vi "Digital_Bridge_3_kart.vi"() -> ()   [LabVIEW 2014] (continued)
                      }
                      frame True {
                        n1874 = local write "Y1 2"(FALSE ("X1 4")) -> ()
                        n1875 = local write "error"(TRUE ("X1 4")) -> ()
                      }
                    }
                    n1876 = local write "10R Yk"(w4993) -> ()
                    n1877 = local write "output 2 y [10R]"(w4992) -> ()
                  }
                  frame True {
                  }
                }
              }
            }
            n1878 = case shown="True" "read x2 y2 2" {
              frame False {
              }
              frame True {
                n1879 = local read "X Range 10R"() -> (w4827:dbl)
                n1880 = call "only_x_and_y_output.vi"("range"=w4827) -> ("cycle 2"=w4831:bool, "range 2"=w4828:dbl, "Output Y"=w4829:dbl, "Output X"=w4830:dbl)  [unwired: 7 in]
                n1881 = case shown="False" w4831 {
                  tunnel: w4830 -> [w4834 _]
                  tunnel: w4829 -> [w4833 _]
                  tunnel: w4828 -> [w4832 w4842]
                  frame False {
                    n1882 = flat-sequence {
                      tunnel: w4834 -> [w4837]
                      tunnel: w4833 -> [w4836]
                      tunnel: w4832 -> [w4835]
                      frame #0 {
                        n1883 = local write "Output X2"(w4837) -> ()
                        n1884 = local write "Output Y2"(w4836) -> ()
                        n1885 = local write "X Range 10R"(w4835) -> ()
                      }
                      frame #1 {
                        n1886 = global write "DB_Global_4_kart-Test.vi" "amplitude 3/0"(0.0) -> ()
                      }
                      frame #2 {
                        n1887 = Wait (ms)(milliseconds to wait=u32 750) -> ()  [unwired: 1 out]
                      }
                      frame #3 {
                        n1888 = local write "result phase 2"(TRUE ("result phase 4")) -> ()
                        n1889 = local write "read x2 y2 2"(FALSE ("output y")) -> ()
                      }
                    }
                  }
                  frame True {
                    n1890 = local write "X Range 10R"(w4842) -> ()
                  }
                }
              }
            }
            n1891 = case shown="True" "IF ELSE X 2" {
              frame False {
              }
              frame True {
                n1892 = local read "input 1 x [10R]"() -> (w5038:dbl)
                n1893 = local read "input 2 x [10R]"() -> (w5039:dbl)
                n1894 = local read "output 1 x [10R]"() -> (w5042:dbl)
                n1895 = local read "result output x [10R]"() -> (w5044:dbl)
                n1896 = local read "output 2 x [10R]"() -> (w5043:dbl)
                n1897 = call "If Else X.vi"("denge degeri"=2.0, "Xk"=w5038, "X(k-1)"=w5039, "output x 1"=w5042, "output x 2"=w5043, "result output x"=w5044) -> ("Output X(k-1)"=w5037:dbl, "Start X"=w5040:bool)  [unwired: 8 in]
                n1898 = local write "10R X(k-1)"(w5037) -> ()
                n1899 = case shown="True" w5040 {
                  frame False {
                  }
                  frame True {
                    n1900 = local read "count meas"() -> (w5045:u16)
                    n1901 = local write "RESET SENS X 2"(TRUE ("START X 4")) -> ()
                    n1902 = local write "IF ELSE X 2"(FALSE ("IF ELSE X 4")) -> ()
                    n1903 = Increment(x=w5045) -> (x+1=w5046:u16)
                    n1904 = local write "count meas"(w5046) -> ()
                  }
                }
              }
            }
            n1905 = case shown="True" "IF ELSE Y 2" {
              frame False {
              }
              frame True {
                n1906 = local read "input 1 y [10R]"() -> (w4953:dbl)
                n1907 = local read "input 2 y [10R]"() -> (w4954:dbl)
                n1908 = local read "output 1 y [10R]"() -> (w4957:dbl)
                n1909 = local read "result output y [10R]"() -> (w4959:dbl)
                n1910 = local read "output 2 y [10R]"() -> (w4958:dbl)
                n1911 = call "If Else Y.vi"("denge degeri"=2.0, "Yk"=w4953, "Y(k-1)"=w4954, "output y 1"=w4957, "output y 2"=w4958, "result output y"=w4959) -> ("Output Y(k-1)"=w4952:dbl, "Start Y"=w4955:bool)  [unwired: 8 in]
                n1912 = local write "10R Y(k-1)"(w4952) -> ()
                n1913 = case shown="True" w4955 {
                  frame False {
                  }
                  frame True {
                    n1914 = local read "count meas"() -> (w4960:u16)
                    n1915 = local write "RESET SENS Y 2"(TRUE ("START X 4")) -> ()
                    n1916 = local write "IF ELSE Y 2"(FALSE ("IF ELSE X 4")) -> ()
                    n1917 = Increment(x=w4960) -> (x+1=w4961:u16)
                    n1918 = local write "count meas"(w4961) -> ()
                  }
                }
              }
            }
            n1919 = case shown="True" "KONTROL X 2" {
              frame False {
              }
              frame True {
                n1920 = local read "Output Denge Kosulu x1_x2"() -> (w4936:dbl[][])
                n1921 = local read "iterasyon 10R"() -> (w4928:dbl)
                n1922 = local read "Manuel/Otomatik"() -> (w4935:enum16{"Manuel", "Otomatik"})
                n1923 = local read "frekans index"() -> (w4929:dbl)
                n1924 = call "Kontrol X.vi"("denge degeri"=2.0, "İterasyon Denge"=w4928, "Denge Kosulu x1_x2"=w4936, "Manuel/Otomatik"=w4935, "frekans index"=w4929) -> ("Denge Seçimi"=w4932:u8, "New İterasyon Denge"=w4931:dbl, "Iterasyon Count Successful"=w4930:dbl, "Start Denge X"=w4933:bool)  [unwired: 7 in]
                n1925 = case shown="True" w4933 {
                  tunnel: w4932 -> [w4948 _]
                  tunnel: w4931 -> [_ _]
                  tunnel: w4930 -> [w4947 _]
                  frame False {
                    n1926 = local write "Iterasyon Successful"(w4947) -> ()
                    n1927 = local write "1R switch"(TRUE ("10R switch")) -> ()
                    n1928 = local write "Denge Seçimi"(w4948) -> ()
                    n1929 = local read "iterasyon 10R"() -> (w4938:dbl)
                    n1930 = local write "KONTROL X 2"(FALSE ("KONTROL X 2")) -> ()
                    n1931 = local write "Boolean 2"(TRUE ("Boolean 4")) -> ()
                    n1932 = Increment(x=w4938) -> (x+1=w4937:dbl)
                    n1933 = local write "iterasyon 10R"(w4937) -> ()
                    n1934 = local read "cycle 10r 1r"() -> (w4940:bool[])
                    n1935 = local write "count meas"(u16 0 ("count meas")) -> ()
                    n1936 = Replace Array Subset(array=w4940, new element=TRUE ("new element/subarray"), index=0) -> (w4941:bool[])
                    n1937 = local write "cycle 10r 1r"(w4941) -> ()
                  }
                  frame True {
                    n1938 = local write "KONTROL X 2"(FALSE ("KONTROL X 2")) -> ()
                    n1939 = local write "count meas"(u16 0 ("count meas")) -> ()
                    n1940 = local write "RESET SENS X 2"(TRUE ("Start Wagner Y")) -> ()
                  }
                }
              }
            }
            n1941 = case shown="True" "result phase 2" {
              frame False {
              }
              frame True {
                n1942 = flat-sequence {
                  tunnel: [w4872] -> w4867
                  tunnel: w4867 -> [w4888]
                  tunnel: [w4888] -> w4866
                  tunnel: w4866 -> [w4893]
                  tunnel: [w4893] -> w4865
                  tunnel: w4865 -> [w4899]
                  frame #0 {
                    # "pi"
                    n1943 = local read "Output X1"() -> (w4871:dbl)
                    n1944 = local read "Output X2"() -> (w4870:dbl)
                    n1945 = local read "Output Y1"() -> (w4869:dbl)
                    n1946 = local read "Output Y2"() -> (w4868:dbl)
                    n1947 = local read "GPIB In"() -> (w4877:refnum<visa-resource-name>)
                    n1948 = call "return phase.vi"("VISA resource name"=w4877) -> ("return phase"=w4873:string)  [unwired: 10 in]
                    n1949 = Fract/Exp String To Number(use system decimal point (T)=FALSE, string=w4873) -> (number=w4875:dbl)  [unwired: 2 in, 1 out]
                    n1950 = formula code="theta = atan((y2-y1)/(x2-x1))*(180/pi)+phase;"("x1"=w4871, "x2"=w4870, "y1"=w4869, "y2"=w4868, "phase"=w4875, "pi"=3.141592653589793) -> ("theta"=w4872:dbl)
                  }
                  frame #1 {
                    n1951 = local read "frekans index"() -> (w4885:dbl)
                    n1952 = local read "Frekanslar"() -> (w4886:dbl[])
                    n1953 = local read "Direnc 1 - Direnc 2"() -> (w4890:u32)
                    n1954 = property on="Default Values Listbox" class="LstBox (strict)"() -> ("Item Names"=w4887:string[])  [unwired: 2 in, 2 out]
                    n1955 = Fract/Exp String To Number(string=w4887) -> (number=w4884:dbl[])  [unwired: 3 in, 1 out]
                    n1956 = local read "Cluster 2"() -> (w4880:T1)
                    n1957 = Index Array(array=w4886, index=w4885) -> (element=w4882:dbl)
                    n1958 = local read "10R F/P Array"() -> (w4891:dbl[][])
                    n1959 = Search 1D Array(1D array=w4884, element=w4882, start index (0)=0) -> (index of element=w4881:i32)
                    n1960 = Increment(x=w4890) -> (x+1=w4889:u32)
                    n1961 = Replace Array Subset(array=w4891, new element=w4888, index (row)=w4889, index (col)=w4881) -> (w4878:dbl[][])
                    n1962 = local write "10R F/P Array"(w4878) -> ()
                    n1963 = Bundle By Name(cluster=w4880, "10R F/P Array"=w4878) -> (w4879:T1)
                    n1964 = local write "Cluster 2"(w4879) -> ()
                  }
                  frame #2 {
                    n1965 = Wait (ms)(milliseconds to wait=u32 250) -> ()  [unwired: 1 out]
                  }
                  frame #3 {
                    w4896 = u16 0 items=["A", "A-B"] ("Input Source (0: A)")
                    n1966 = local read "GPIB In"() -> (w4895:refnum<visa-resource-name>)
                    n1967 = Number To Fractional String(number=w4899) -> (F-format string=w4900:string)  [unwired: 3 in]
                    n1968 = Search and Replace String(input string=w4900, search string=",", replace string="." ("replace string (\"\")")) -> (result string=w4894:string)  [unwired: 5 in, 3 out]
                    n1969 = call "reference phase.vi"("Reference Phase (0.000 degrees)"=w4894, "VISA resource name"=w4895) -> ("error out"=w4897:errorcluster, "VISA resource name out"=w4898:refnum<visa-resource-name>)  [unwired: 8 in]
                    n1970 = call "input source.vi"("error in (no error)"=w4897, "Input Source (0: A)"=w4896, "VISA resource name"=w4898) -> ()  [unwired: 7 in, 2 out]
                  }
                  frame #4 {
                    n1971 = local write "Contiune 10R"(TRUE ("Contiune Wagner")) -> ()
                    n1972 = local write "result phase 2"(FALSE ("result phase 4")) -> ()
                  }
                }
              }
            }
            n1973 = case shown="True" "KONTROL Y 2" {
              frame False {
              }
              frame True {
                n1974 = local read "Outpu Denge Kosulu y1_y2"() -> (w5021:dbl[][])
                n1975 = local read "iterasyon 10R"() -> (w5013:dbl)
                n1976 = local read "Manuel/Otomatik"() -> (w5020:enum16{"Manuel", "Otomatik"})
                n1977 = local read "frekans index"() -> (w5014:dbl)
                n1978 = call "Kontrol Y.vi"("denge degeri"=2.0, "İterasyon Denge"=w5013, "Denge Kosulu y1_y2"=w5021, "Manuel/Otomatik"=w5020, "frekans index"=w5014) -> ("Denge Seçimi"=w5017:u8, "New İterasyon Denge"=w5016:dbl, "Iterasyon Count Successful"=w5015:dbl, "Start Denge Y"=w5018:bool)  [unwired: 7 in]
                n1979 = case shown="True" w5018 {
                  tunnel: w5017 -> [w5033 _]
                  tunnel: w5016 -> [_ _]
                  tunnel: w5015 -> [w5032 _]
                  frame False {
                    n1980 = local read "iterasyon 10R"() -> (w5023:dbl)
                    n1981 = local write "Iterasyon Successful"(w5032) -> ()
                    n1982 = local write "Denge Seçimi"(w5033) -> ()
                    n1983 = local write "1R switch"(TRUE ("10R switch")) -> ()
                    n1984 = local write "KONTROL Y 2"(FALSE ("KONTROL Y 2")) -> ()
                    n1985 = local write "Boolean 2"(TRUE ("Boolean 4")) -> ()
                    n1986 = Increment(x=w5023) -> (x+1=w5022:dbl)
                    n1987 = local write "iterasyon 10R"(w5022) -> ()
                    n1988 = local read "cycle 10r 1r"() -> (w5025:bool[])
                    n1989 = local write "count meas"(u16 0 ("count meas")) -> ()
                    n1990 = Replace Array Subset(array=w5025, new element=TRUE ("new element/subarray"), index=0) -> (w5026:bool[])
                    n1991 = local write "cycle 10r 1r"(w5026) -> ()
                  }
                  frame True {
                    n1992 = local write "KONTROL Y 2"(FALSE ("KONTROL Y 2")) -> ()
                    n1993 = local write "count meas"(u16 0 ("count meas")) -> ()
                    n1994 = local write "RESET SENS Y 2"(TRUE ("Start Wagner Y")) -> ()
                  }
                }
              }
            }
          }
          frame 3 {
            # "Bu bölümde, ilgili denge durumunun dengede olup olmadığı kontrol edilir.\n\nEğer denge sağlanmışsa, program doğrudan bir sonraki denge aşamasına geçer.\n\nAyrıca, tüm dengeler başarıyla tamamlanmış ve belirlenen ölçüm sayısına ulaşılmışsa, veriler bu alt program (subVI) aracılığıyla Excel dosyasına aktarılır."
            # "Bu bölümün temel amacı, ölçüm aralığını (range) artırmaktır. Program, cihazdan gelen X ve Y değerlerini okuyarak bu değerlerin belirlenen aralık içinde olup olmadığını kontrol eder. \n\nEğer değerler aralık dışındaysa, aralık tekrar artırılır ve ölçüm yeniden yapılır. \n\nAyrıca, bu süreçte input ve output değerleri global değişkenlere kaydedilir. Çünkü sonraki turda, bu kaydedilen değerler farklı bir ölçüm aralığında eğim hesaplaması için kullanılacaktır."
            # "Bu bölümde, sıfırlanacak değer cihazdan okunur. Eğer okunan değer denge koşulunu sağlıyorsa, program Kontrol Y Case’ine geçer. \n\nAncak denge koşulu sağlanmazsa, program if-else yapısına yönlendirilir ve buna göre işlem devam eder."
            # "Bu bölümde, cihaza ikinci input değeri uygulanır ve karşılık gelen output değeri okunur. Daha sonra, hem input hem de output değerleri bir formüle yerleştirilir. Bu formül sayesinde, cihazın 0’a eşitleyeceği (sıfırlayacağı) yeni bir input değeri hesaplanır ve bu değer cihaza uygulanır."
            # "Bu bölümde ilk olarak giriş (input) değeri sisteme uygulanır. Eğer program ilk kez çalıştırılıyorsa, global input üzerinden belirlenen ilk değer (genellikle 0 V) kullanılır. \n\nArdından, cihazdan X değerleri okunur. Bu işlem 10 kez tekrarlanır ve elde edilen ölçümlerin ortalaması alınarak bir sonuç değeri elde edilir. Bu ortalama değer, daha sonra yapılacak işlemlerde kullanılmak üzere saklanır. Özellikle, formül içinde X değerini sıfırlamak için bu bilgiye ihtiyaç duyulur. \n\nEğer girilen input değeri 8 V’tan büyükse, bu durum sistem için güvenli olmayabileceğinden program hata (error) verir ve işlemi durdurur."
            # "Auto Phase, Read X1 Y1, Read X2 Y2, Result Phase: \n\nBu bölümler genel olarak faz ölçümü işlemini gerçekleştirir. \n\nİlk olarak, faz değeri 0’a sıfırlanır. Ardından, global input üzerinden belirlenen range (ölçüm aralığı) değeri uygulanır. Bu işlemden sonra yine global input’ta tanımlanmış olan: \n\nInput 1 verilir ve okuma yapılır (Read X1 Y1) \n\nInput 2 verilir ve okuma yapılır (Read X2 Y2) \n\nBu iki ölçüm sonucuna göre faz değeri bir formül yardımıyla hesaplanır. Elde edilen bu yeni faz değeri, ilgili F/P (frekans/faz) dizisine aktarılır. \n\nBu işlemler, sistemin doğru fazla çalışmasını sağlamak ve sonraki işlemlerde bu bilgiyi referans olarak kullanmak için gerçekleştirilir."
            # "Bu bölümde, Y değerinin dengelendiği kabul edilerek, şimdi sıra X değerinin dengede olup olmadığını kontrol etmeye gelir. \n\nEğer X de dengedeyse, program bir sonraki işlem için ilgili switch case’i aktif eder. \n\nAncak Y dengede değilse, program X’i dengelemeye yönelik işlemlere yönlendirilir."
            # "Bu bölümde, X değerinin dengelendiği kabul edilerek, şimdi sıra Y değerinin dengede olup olmadığını kontrol etmeye gelir. \n\nEğer Y de dengedeyse, program bir sonraki işlem için ilgili switch case’i aktif eder. \n\nAncak Y dengede değilse, program Y’yi dengelemeye yönelik işlemlere yönlendirilir."
            # "X1 3 ile benzer görevi üstleniyor sadece değerler Y oluyor"
            # "IF ELSE X 3 ile benzer görevi üstleniyor sadece değerler Y oluyor"
            # "X 3 ile benzer görevi üstleniyor sadece değerler Y oluyor"
            # "Range Kontrol X 3 ile benzer görevi üstleniyor sadece değerler Y oluyor"
            # "Bu bölümde, daha önce iterasyon (tekrarlama) yapılıp yapılmadığına bakılarak, programın hangi yöne devam edeceğine karar verilir. \n\nEğer gerekli ise, range kontrolü (ölçüm aralığının uygunluğu) yapılır veya sensitivity ayarlama (cihazın duyarlılığını belirleme) bölümlerine yönlendirilir. Bu sayede sistem, ölçüm koşullarına en uygun şekilde ayarlanarak doğru ve güvenilir sonuçlar elde edilmesi sağlanır."
            # "Bu bölümde, daha önce belirlenen F/P dizilerindeki (frekans/faz değerleri) faz bilgileri, mevcut frekansa göre uygulanır. Ardından, ilgili denge koşulunun daha önce gerçekleştirilip gerçekleştirilmediği kontrol edilir. \nEğer bu denge daha önce sağlanmamışsa, program uygun faz ayarlamasını yapar. Ancak denge daha önce zaten kurulmuşsa, faz ayarı yapılmadan işleme devam edilir. Bu sayede gereksiz tekrarların önüne geçilmiş olur."
            # "Bu bölümde öncelikle, sistemin kaç kez ölçüm yaptığına işaret eden meas number (ölçüm sayısı) kontrol edilir. \nEğer bu sayı 6’dan büyükse (bu sınır kullanıcı tarafından belirlenmiştir ve değiştirilebilir), program hata verir ve reset values adlı bölüme yönlenir. Bu durum, sistemin çok fazla başarısız deneme yapmasını engellemek içindir. \nEğer ölçüm sayısı 6’dan küçükse, program global bir değişken olan sensitivity (duyarlılık) değerini ayarlar ve ardından işlemlere devam etmek üzere Start X bölümüne geçer."
            # "Bu bölümde, ölçüm için gerekli olan giriş (input) değerleri sisteme girilir. Girişler tamamlandıktan sonra program, ölçüm işlemini başlatmak üzere X adlı bölüme yönlendirilir. Bu adım, ölçüm sürecinin fiilen başlatıldığı ilk noktadır."
            # "Pass subvi girmeden önce doğru range miyiz değil miyiz ölçüyor, değil ise +2 üst kademeye gidiyor"
            # "Start 1R X ile benzer görevi üstleniyor sadece değerler Y oluyor"
            # "Reset Sens X 3 ile benzer görevi üstleniyor sadece değerler Y oluyor"
            # "Start X 3 ile benzer görevi üstleniyor sadece değerler Y oluyor"
            # "Bu bölüm, iterasyona (tekrarlamalı işleme) bağlı olarak Reserve ayarının maksimumda mı yoksa minimumda mı olacağını belirler. Aynı zamanda, ölçüm sürecinin başlangıcında kullanılacak olan sensitivity  değerleri de bu bölümde ayarlanır. Bu ayarlar, ölçüm sırasında cihazın hassasiyetini ve çalışma aralığını doğru şekilde belirlemek için gereklidir."
            # "1R"
            n1995 = case shown="True" "Start 1R Y" {
              frame False {
              }
              frame True {
                n1996 = flat-sequence {
                  frame #0 {
                    w5867 = u16 0 items=["A", "A-B"] ("Input Source (0: A)")
                    n1997 = local read "frekans index"() -> (w5861:dbl)
                    n1998 = local read "Frekanslar"() -> (w5862:dbl[])
                    n1999 = local read "Direnc 1 - Direnc 2"() -> (w5864:u32)
                    n2000 = local read "1R F/P Array"() -> (w5865:dbl[][])
                    n2001 = Index Array(array=w5862, index=w5861) -> (element=w5863:dbl)
                    n2002 = call "get_phase_element.vi"("index r"=w5864, "hz"=w5863, "Array"=w5865) -> ("element"=w5857:dbl)  [unwired: 8 in]
                    n2003 = Number To Fractional String(number=w5857) -> (F-format string=w5858:string)  [unwired: 3 in]
                    n2004 = Search and Replace String(input string=w5858, search string=",", replace string="." ("replace string (\"\")")) -> (result string=w5856:string)  [unwired: 5 in, 3 out]
                    n2005 = local read "GPIB In"() -> (w5866:refnum<visa-resource-name>)
                    n2006 = call "reference phase.vi"("Reference Phase (0.000 degrees)"=w5856, "VISA resource name"=w5866) -> ("error out"=w5868:errorcluster, "VISA resource name out"=w5869:refnum<visa-resource-name>)  [unwired: 8 in]
                    n2007 = call "input source.vi"("error in (no error)"=w5868, "Input Source (0: A)"=w5867, "VISA resource name"=w5869) -> ()  [unwired: 7 in, 2 out]
                  }
                  frame #1 {
                    n2008 = local write "Boolean 3"(FALSE ("Boolean 4")) -> ()
                    n2009 = local write "Start 1R Y"(FALSE ("START Y 6")) -> ()
                    n2010 = local write "RESET SENS Y 3"(TRUE ("START X")) -> ()
                  }
                }
              }
            }
            n2011 = case shown="True" "RESET SENS Y 3" {
              frame False {
              }
              frame True {
                n2012 = local read "count meas"() -> (w5836:u16)
                n2013 = local read "iterasyon 1R"() -> (w5834:dbl)
                n2014 = Greater?(x=w5836, y=u16 8) -> (0:w5833:bool)
                n2015 = Greater?(x=w5834, y=10.0) -> (0:w5832:bool)
                n2016 = Or(x=w5833, y=w5832) -> (x .or. y?=w5831:bool)
                n2017 = case shown="True" w5831 {
                  frame False {
                    n2018 = flat-sequence {
                      frame #0 {
                        n2019 = global read "show_sensitivity.vi" "show sensitivity (1R  y)"() -> (w5838:dbl)
                        n2020 = local read "GPIB In"() -> (w5839:refnum<visa-resource-name>)
                        n2021 = call "get_sensitivity.vi"("input 1"=w5838, "SR850 GPIB In"=w5839) -> ()  [unwired: 8 in, 2 out]
                      }
                      frame #1 {
                        n2022 = Wait (ms)(milliseconds to wait=u32 500) -> ()  [unwired: 1 out]
                      }
                      frame #2 {
                        n2023 = local write "RESET SENS Y 3"(FALSE ("RESET SENS X")) -> ()
                        n2024 = local write "START Y 3"(TRUE ("START X 4")) -> ()
                      }
                    }
                  }
                  frame True {
                    n2025 = local read "iterasyon 1R"() -> (w5845:dbl)
                    n2026 = Greater?(x=w5845, y=10.0) -> (0:w5843:bool)
                    n2027 = case shown="False" w5843 {
                      frame False {
                        n2028 = flat-sequence {
                          frame #0 {
                            n2029 = local write "RESET SENS Y 3"(FALSE ("Start 10R X")) -> ()
                            n2030 = local write "İterasyon X 3"(0.0 ("İterasyon X 3")) -> ()
                            n2031 = local write "count meas"(u16 9 ("count meas")) -> ()
                          }
                          frame #1 {
                            n2032 = local write "reset values"(TRUE ("Start 10R X")) -> ()
                            n2033 = local write "error"(TRUE ("Start 10R X")) -> ()
                          }
                        }
                      }
                      frame True {
                        n2034 = flat-sequence {
                          frame #0 {
                            n2035 = local write "RESET SENS Y 3"(FALSE ("Start 10R X")) -> ()
                            n2036 = local write "İterasyon X 3"(0.0 ("İterasyon X 3")) -> ()
                            n2037 = local write "count meas"(u16 10 ("count meas")) -> ()
                          }
                          frame #1 {
                            n2038 = local write "reset values"(TRUE ("Start 10R X")) -> ()
                            n2039 = local write "error"(TRUE ("Start 10R X")) -> ()
                          }
                        }
                      }
                    }
                  }
                }
              }
            }
            n2040 = case shown="True" "START Y 3" {
              frame False {
              }
              frame True {
                n2041 = flat-sequence {
                  frame #0 {
                    n2042 = local read "1R Y(k-1)"() -> (w5874:dbl)
                    n2043 = local read "1R Yk"() -> (w5873:dbl)
                    n2044 = local write "input 1 y [1R]"(w5873) -> ()
                    n2045 = local write "input 2 y [1R]"(w5874) -> ()
                    n2046 = global write "DB_Global_4_kart-Test.vi" "phase 3/1"(w5873) -> ()
                  }
                  frame #1 {
                    n2047 = Wait (ms)(milliseconds to wait=u32 500) -> ()  [unwired: 1 out]
                  }
                  frame #2 {
                    n2048 = local write "START Y 3"(FALSE ("START X")) -> ()
                    n2049 = local write "Y 3"(TRUE ("START X")) -> ()
                  }
                }
              }
            }
            n2050 = case shown="True" "Start 1R X" {
              frame False {
              }
              frame True {
                n2051 = flat-sequence {
                  frame #0 {
                    w5774 = u16 0 items=["A", "A-B"] ("Input Source (0: A)")
                    n2052 = local read "frekans index"() -> (w5769:dbl)
                    n2053 = local read "Frekanslar"() -> (w5770:dbl[])
                    n2054 = local read "Direnc 1 - Direnc 2"() -> (w5771:u32)
                    n2055 = local read "1R F/P Array"() -> (w5772:dbl[][])
                    n2056 = Index Array(array=w5770, index=w5769) -> (element=w5768:dbl)
                    n2057 = call "get_phase_element.vi"("index r"=w5771, "hz"=w5768, "Array"=w5772) -> ("element"=w5764:dbl)  [unwired: 8 in]
                    n2058 = Number To Fractional String(number=w5764) -> (F-format string=w5767:string)  [unwired: 3 in]
                    n2059 = local read "GPIB In"() -> (w5773:refnum<visa-resource-name>)
                    n2060 = Search and Replace String(input string=w5767, search string=",", replace string="." ("replace string (\"\")")) -> (result string=w5763:string)  [unwired: 5 in, 3 out]
                    n2061 = call "reference phase.vi"("Reference Phase (0.000 degrees)"=w5763, "VISA resource name"=w5773) -> ("error out"=w5775:errorcluster, "VISA resource name out"=w5776:refnum<visa-resource-name>)  [unwired: 8 in]
                    n2062 = call "input source.vi"("error in (no error)"=w5775, "Input Source (0: A)"=w5774, "VISA resource name"=w5776) -> ()  [unwired: 7 in, 2 out]
                  }
                  frame #1 {
                    n2063 = local read "1 or 10"() -> (w5791:i32)
                    n2064 = local read "İterasyon X 3"() -> (w5787:dbl)
                    n2065 = local read "frekans index"() -> (w5786:dbl)
                    n2066 = local read "control hz array"() -> (w5782:dbl[][])
                    n2067 = Greater?(x=w5787, y=0.0) -> (0:w5788:bool)
                    n2068 = call "change2d.vi"("reset(default false)"=FALSE, "index (col)"=w5786, "index (row)"=2, "read/write(T/F)"=TRUE, "2D Array"=w5782) -> ("result count"=w5781:dbl)  [unwired: 5 in, 1 out]
                    n2069 = Equal?(x=w5791, y=1) -> (x = y?=w5789:bool)
                    n2070 = Or(x=w5788, y=w5789) -> (x .or. y?=w5778:bool)
                    n2071 = local read "set"() -> (w5780:u16)
                    n2072 = Equal?(x=w5781, y=w5780) -> (x = y?=w5779:bool)
                    n2073 = Or(x=w5778, y=w5779) -> (x .or. y?=w5777:bool)
                    n2074 = case shown="True" w5777 {
                      frame False {
                        n2075 = local write "auto phase 1R"(TRUE ("auto phase 10R")) -> ()
                        n2076 = local write "Start 1R X"(FALSE ("auto phase 10R")) -> ()
                      }
                      frame True {
                        n2077 = local write "Contiune 1R"(TRUE) -> ()
                        n2078 = local write "Start 1R X"(FALSE ("START WAGNER")) -> ()
                      }
                    }
                  }
                }
              }
            }
            n2079 = case shown="True" "1R switch" {
              frame False {
              }
              frame True {
                n2080 = flat-sequence {
                  frame #0 {
                    n2081 = local read "iterasyon 1R"() -> (w5797:dbl)
                    n2082 = Equal?(x=w5797, y=0.0) -> (x = y?=w5798:bool)
                    n2083 = case shown="True" w5798 {
                      frame False {
                      }
                      frame True {
                        n2084 = local read "1 or 10"() -> (w5800:i32)
                        n2085 = case shown="1" w5800 {
                          frame 0, Default {
                          }
                          frame 1 {
                            n2086 = local write "iterasyon 1R"(1.0 ("iterasyon WAGNER")) -> ()
                          }
                        }
                      }
                    }
                  }
                  frame #1 {
                    n2087 = local read "iterasyon 1R"() -> (w5803:dbl)
                    n2088 = Greater?(x=w5803, y=0.0) -> (0:w5802:bool)
                    n2089 = case shown="True" w5802 {
                      frame False {
                        n2090 = local read "Reserve 1R"() -> (w5806:u16)
                        n2091 = case shown="0, Default" w5806 {
                          tunnel: ["0" ("Reserve(MAX-MIN)") "1" ("Reserve(MAX-MIN)") "2" ("Reserve(MAX-MIN)")] -> w5805
                          frame 0, Default {
                          }
                          frame 1 {
                          }
                          frame 2 {
                          }
                        }
                        n2092 = local read "GPIB In"() -> (w5807:refnum<visa-resource-name>)
                        n2093 = call "Reserve.vi"("Reserve(MAX-MIN)"=w5805, "VISA resource name"=w5807) -> ()  [unwired: 8 in, 2 out]
                      }
                      frame True {
                        n2094 = local read "GPIB In"() -> (w5812:refnum<visa-resource-name>)
                        n2095 = call "Reserve.vi"("Reserve(MAX-MIN)"="0", "VISA resource name"=w5812) -> ()  [unwired: 8 in, 2 out]
                      }
                    }
                  }
                  frame #2 {
                    n2096 = Wait (ms)(milliseconds to wait=u32 500) -> ()  [unwired: 1 out]
                  }
                  frame #3 {
                    w5815 = u16 1 items=["Wagner", "Ground"] ("Switch")
                    w5816 = u16 3 items=["Open All", "Ana Denge", "10R", "1R"] ("Ring")
                    n2097 = call "mux1.vi"("Ring"=w5816) -> ("error out"=w5817:errorcluster)  [unwired: 9 in]
                    n2098 = property on="Tab Control" class="TabCtl (strict)"("Value"=T4."1R" ("Tab Control")) -> ()  [unwired: 2 in, 2 out]
                    n2099 = call "mux2.vi"("Switch"=w5815, "error in (no error)"=w5817) -> ()  [unwired: 6 in, 1 out]
                  }
                  frame #4 {
                    n2100 = Wait (ms)(milliseconds to wait=u32 1000) -> ()  [unwired: 1 out]
                  }
                  frame #5 {
                    n2101 = local read "İterasyon X 3"() -> (w5825:dbl)
                    n2102 = local read "1 or 10"() -> (w5822:i32)
                    n2103 = Equal?(x=w5822, y=1) -> (x = y?=w5821:bool)
                    n2104 = Greater?(x=w5825, y=0.0) -> (0:w5820:bool)
                    n2105 = Or(x=w5820, y=w5821) -> (x .or. y?=w5819:bool)
                    n2106 = case shown="False" w5819 {
                      frame False {
                        n2107 = local read "X Range 1R"() -> (w5827:dbl)
                        n2108 = local read "Y Range 1R"() -> (w5826:dbl)
                        n2109 = global write "show_sensitivity.vi" "show sensitivity (1R  x)"(w5827) -> ()
                        n2110 = global write "show_sensitivity.vi" "show sensitivity (1R  y)"(w5826) -> ()
                      }
                      frame True {
                        w5828 = 16.0 ("Max. Hassasiyet")
                        n2111 = global write "show_sensitivity.vi" "show sensitivity (1R  x)"(w5828) -> ()
                        n2112 = global write "show_sensitivity.vi" "show sensitivity (1R  y)"(w5828) -> ()
                      }
                    }
                  }
                  frame #6 {
                    n2113 = local write "Start 1R X"(TRUE ("START WAGNER")) -> ()
                    n2114 = local write "1R switch"(FALSE ("wagner switch")) -> ()
                  }
                }
              }
            }
            n2115 = case shown="True" "RESET SENS X 3" {
              frame False {
              }
              frame True {
                n2116 = local read "count meas"() -> (w5884:u16)
                n2117 = local read "iterasyon 1R"() -> (w5881:dbl)
                n2118 = Greater?(x=w5884, y=u16 8) -> (0:w5880:bool)
                n2119 = Greater?(x=w5881, y=5.0) -> (0:w5879:bool)
                n2120 = Or(x=w5880, y=w5879) -> (x .or. y?=w5878:bool)
                n2121 = case shown="True" w5878 {
                  frame False {
                    n2122 = flat-sequence {
                      frame #0 {
                        n2123 = global read "show_sensitivity.vi" "show sensitivity (1R  x)"() -> (w5885:dbl)
                        n2124 = local read "GPIB In"() -> (w5886:refnum<visa-resource-name>)
                        n2125 = call "get_sensitivity.vi"("input 1"=w5885, "SR850 GPIB In"=w5886) -> ()  [unwired: 8 in, 2 out]
                      }
                      frame #1 {
                        n2126 = Wait (ms)(milliseconds to wait=u32 500) -> ()  [unwired: 1 out]
                      }
                      frame #2 {
                        n2127 = local write "RESET SENS X 3"(FALSE ("RESET SENS X")) -> ()
                        n2128 = local write "START X 3"(TRUE ("START X 4")) -> ()
                      }
                    }
                  }
                  frame True {
                    n2129 = local read "iterasyon 1R"() -> (w5892:dbl)
                    n2130 = Greater?(x=w5892, y=5.0) -> (0:w5890:bool)
                    n2131 = case shown="False" w5890 {
                      frame False {
                        n2132 = flat-sequence {
                          frame #0 {
                            n2133 = local write "count meas"(u16 9 ("count meas")) -> ()
                            n2134 = local write "İterasyon X 3"(0.0 ("İterasyon X 3")) -> ()
                            n2135 = local write "RESET SENS X 3"(FALSE ("Start 10R X")) -> ()
                          }
                          frame #1 {
                            n2136 = local write "reset values"(TRUE ("Start 10R X")) -> ()
                            n2137 = local write "error"(TRUE ("Start 10R X")) -> ()
                          }
                        }
                      }
                      frame True {
                        n2138 = flat-sequence {
                          frame #0 {
                            n2139 = local write "count meas"(u16 10 ("count meas")) -> ()
                            n2140 = local write "İterasyon X 3"(0.0 ("İterasyon X 3")) -> ()
                            n2141 = local write "RESET SENS X 3"(FALSE ("Start 10R X")) -> ()
                          }
                          frame #1 {
                            n2142 = local write "reset values"(TRUE ("Start 10R X")) -> ()
                            n2143 = local write "error"(TRUE ("Start 10R X")) -> ()
                          }
                        }
                      }
                    }
                  }
                }
              }
            }
            n2144 = case shown="True" "START X 3" {
              frame False {
              }
              frame True {
                n2145 = flat-sequence {
                  frame #0 {
                    n2146 = local read "1R X(k-1)"() -> (w5904:dbl)
                    n2147 = local read "1R Xk"() -> (w5903:dbl)
                    n2148 = global write "DB_Global_4_kart-Test.vi" "amplitude 3/1"(w5903) -> ()
                    n2149 = local write "input 1 x [1R]"(w5903) -> ()
                    n2150 = local write "input 2 x [1R]"(w5904) -> ()
                  }
                  frame #1 {
                    n2151 = Wait (ms)(milliseconds to wait=u32 500) -> ()  [unwired: 1 out]
                  }
                  frame #2 {
                    n2152 = local write "START X 3"(FALSE ("START X 4")) -> ()
                    n2153 = local write "X 3"(TRUE ("START X")) -> ()
                  }
                  frame #3 {
                  }
                }
              }
            }
            n2154 = case shown="True" "Optimum Range 3" {
              frame False {
              }
              frame True {
                n2155 = flat-sequence {
                  frame #0 {
                    n2156 = global read "show_sensitivity.vi" "show sensitivity (1R  x)"() -> (w5417:dbl)
                    n2157 = local read "GPIB In"() -> (w5416:refnum<visa-resource-name>)
                    n2158 = call "get_sensitivity.vi"("input 1"=w5417, "SR850 GPIB In"=w5416) -> ()  [unwired: 8 in, 2 out]
                  }
                  frame #1 {
                    n2159 = call "set optimum range.vi"("denge degeri"=3.0) -> ("ok"=w5418:bool)  [unwired: 14 in]
                    n2160 = case shown="True" w5418 {
                      frame False {
                      }
                      frame True {
                        n2161 = local write "Optimum Range 3"(FALSE ("Optimum Range 1")) -> ()
                        n2162 = local write "PASS 1R"(TRUE ("PASS 1R")) -> ()
                      }
                    }
                  }
                }
              }
            }
            n2163 = case shown="True" "Contiune 1R" {
              frame False {
              }
              frame True {
                n2164 = local read "1 or 10"() -> (w5472:i32)
                n2165 = local read "frekans index"() -> (w5471:dbl)
                n2166 = local read "control hz array"() -> (w5467:dbl[][])
                n2167 = call "change2d.vi"("reset(default false)"=FALSE, "index (col)"=w5471, "index (row)"=2, "read/write(T/F)"=TRUE, "2D Array"=w5467) -> ("result count"=w5466:dbl)  [unwired: 5 in, 1 out]
                n2168 = local read "iterasyon 1R"() -> (w5476:dbl)
                n2169 = local read "set"() -> (w5465:u16)
                n2170 = case shown="1" w5472 {
                  tunnel: [FALSE TRUE] -> w5473
                  frame 10, Default {
                  }
                  frame 1 {
                  }
                }
                n2171 = Equal?(x=w5466, y=w5465) -> (x = y?=w5464:bool)
                n2172 = Greater?(x=w5476, y=0.0) -> (0:w5474:bool)
                n2173 = Or(x=w5474, y=w5473) -> (x .or. y?=w5463:bool)
                n2174 = Or(x=w5463, y=w5464) -> (x .or. y?=w5462:bool)
                n2175 = case shown="True" w5462 {
                  frame False {
                    n2176 = local write "RESET SENS X 3"(TRUE ("START X")) -> ()
                    n2177 = local write "Contiune 1R"(FALSE ("START WAGNER")) -> ()
                    n2178 = local write "Boolean 3"(FALSE ("Boolean 4")) -> ()
                  }
                  frame True {
                    n2179 = local write "Optimum Range 3"(TRUE ("START X")) -> ()
                    n2180 = local write "Contiune 1R"(FALSE ("Boolean 4")) -> ()
                    n2181 = local write "Boolean 3"(FALSE ("Boolean 4")) -> ()
                  }
                }
              }
            }
            n2182 = case shown="True" "PASS 1R" {
              frame False {
              }
              frame True {
                n2183 = flat-sequence {
                  tunnel: [w5664] -> w5654
                  tunnel: [w5663] -> w5653
                  tunnel: [w5662] -> w5652
                  tunnel: [w5661] -> w5651
                  tunnel: [w5660] -> w5650
                  tunnel: [w5659] -> w5649
                  tunnel: [w5658] -> w5648
                  tunnel: w5654 -> [w5726]
                  tunnel: w5653 -> [w5725]
                  tunnel: w5652 -> [w5724]
                  tunnel: w5651 -> [w5723]
                  tunnel: w5650 -> [w5722]
                  tunnel: w5649 -> [w5721]
                  tunnel: w5648 -> [w5720]
                  frame #0 {
                    n2184 = Wait (ms)(milliseconds to wait=u32 500) -> ()  [unwired: 1 out]
                  }
                  frame #1 {
                    n2185 = local read "Other Array"() -> (w5692:dbl[])
                    n2186 = for {
                      N: 7 -> [_]
                      shift-right: [w5709] -> w5695
                      shift-left: w5692 -> [w5712]
                      i -> [w5711]
                      n2187 = case shown="6" w5711 {
                        tunnel: [3.0 ("iterasyon WAGNER") w5714 w5715 w5716 w5717 w5718 w5719] -> w5710
                        frame 0, Default {
                        }
                        frame 1 {
                          n2188 = local read "Iterasyon Successful"() -> (w5714:dbl)
                        }
                        frame 2 {
                          n2189 = local read "Direnc 1 - Direnc 2"() -> (w5715:u32)
                        }
                        frame 3 {
                          n2190 = local read "olcum"() -> (w5716:u16)
                        }
                        frame 4 {
                          n2191 = local read "set"() -> (w5717:u16)
                        }
                        frame 5 {
                          n2192 = local read "frekans index"() -> (w5718:dbl)
                        }
                        frame 6 {
                          n2193 = local read "iterasyon 1R"() -> (w5719:dbl)
                        }
                      }
                      n2194 = Replace Array Subset(array=w5712, new element=w5710, index=w5711) -> (w5709:dbl[])
                    }
                    n2195 = local read "Output Denge Kosulu x2_y2"() -> (w5697:dbl[][])
                    n2196 = local read "Output Denge Kosulu x1_x2"() -> (w5678:dbl[][])
                    n2197 = control-ref of="Default Values Listbox"() -> (w5682:refnum<vi>)
                    n2198 = local read "Outpu Denge Kosulu y1_y2"() -> (w5677:dbl[][])
                    n2199 = local read "Frekanslar"() -> (w5657:dbl[])
                    n2200 = local read "Cluster"() -> (w5680:T2)
                    n2201 = local read "Cluster 2"() -> (w5679:T1)
                    n2202 = Array Size(array=w5657) -> (size(s)=w5656:i32)
                    n2203 = call "merge_x_y.vi"("frekans size"=w5656, "y1_y2"=w5677, "x1_x2"=w5678) -> ("x1_x2_y1_y2"=w5676:dbl[][])  [unwired: 8 in]
                    n2204 = local read "default values"() -> (w5696:T3)
                    n2205 = local read "input values"() -> (w5681:dbl[])
                    n2206 = local read "Sheet name"() -> (w5693:string)
                    n2207 = local read "Other Boolean Array"() -> (w5691:bool[])
                    n2208 = for {
                      N: 5 -> [_]
                      shift-right: [w5700] -> w5694
                      shift-left: w5691 -> [w5703]
                      i -> [w5702]
                      n2209 = case shown="1" w5702 {
                        tunnel: [FALSE FALSE FALSE FALSE FALSE] -> w5701
                        frame 0, Default {
                        }
                        frame 1 {
                        }
                        frame 2 {
                        }
                        frame 3 {
                        }
                        frame 4 {
                        }
                      }
                      n2210 = Replace Array Subset(array=w5703, new element=w5701, index=w5702) -> (w5700:bool[])
                    }
                    n2211 = call "Pass.vi"("Other Array"=w5695, "Other Boolean Array"=w5694, "Denge Kosulu x2_y2"=w5697, "LstBox Refnum"=w5682, "Cluster"=w5680, "F/P Array Cluster"=w5679, "Sheet name"=w5693, "default values"=w5696, "x1_x2_y1_y2"=w5676, "input values"=w5681) -> ("output values"=w5675:dbl[], "Output Other Boolean Array"=w5688:bool[], "Output Cluster"=w5674:T2, "Output F/P Array Cluster"=w5670:T1, "output default values"=w5690:T11, "Output Iterasyon Successful"=w5689:dbl, "Denge Seçimi"=w5662:u8, "end time"=w5660:string)  [unwired: 1 in, 1 out]
                    n2212 = Unbundle By Name(w5674) -> ("F Values Array"=w5673:dbl[][], "control hz array"=w5672:dbl[][], "extra default values"=w5671:dbl[][])
                    n2213 = Unbundle By Name(w5670) -> ("AD F/P Array"=w5669:dbl[][], "10R F/P Array"=w5668:dbl[][], "1R F/P Array"=w5667:dbl[][], "Wagner F/P Array"=w5666:dbl[][], "Kelvin F/P Array"=w5665:dbl[][])
                    n2214 = local write "input values"(w5675) -> ()
                    n2215 = local write "AD F/P Array"(w5669) -> ()
                    n2216 = local write "10R F/P Array"(w5668) -> ()
                    n2217 = local write "1R F/P Array"(w5667) -> ()
                    n2218 = local write "Wagner F/P Array"(w5666) -> ()
                    n2219 = local write "Kelvin F/P Array"(w5665) -> ()
                    n2220 = local write "F Values Array"(w5673) -> ()
                    n2221 = local write "control hz array"(w5672) -> ()
                    n2222 = local write "extra default values"(w5671) -> ()
                    n2223 = local write "default values"(w5690) -> ()
                    n2224 = local write "Iterasyon Successful"(w5689) -> ()
                    n2225 = Index Array(array=w5688, index #1=0 ("index"), index #2=1 ("index"), index #3=2 ("index"), index #4=3 ("index"), index #5=4 ("index")) -> (element #1=w5664:bool, element #2=w5663:bool, element #3=w5661:bool, element #4=w5659:bool, element #5=w5658:bool)
                  }
                  frame #2 {
                    n2226 = case shown="True" w5720 {
                      frame False {
                      }
                      frame True {
                        n2227 = local write "RESET SENS Y 3"(TRUE ("RESET SENS Y 4")) -> ()
                        n2228 = local write "PASS 1R"(FALSE ("PASS 1R")) -> ()
                      }
                    }
                    n2229 = case shown="True" w5726 {
                      frame False {
                      }
                      frame True {
                        n2230 = local write "reset values"(TRUE ("reset values")) -> ()
                        n2231 = local write "PASS 1R"(FALSE ("PASS 1R")) -> ()
                        n2232 = local write "pass hz"(TRUE ("pass hz")) -> ()
                        n2233 = local write "Boolean 3"(TRUE ("Boolean 4")) -> ()
                      }
                    }
                    n2234 = case shown="True" w5725 {
                      tunnel: w5724 -> [_ w5735]
                      frame False {
                      }
                      frame True {
                        n2235 = local read "cycle 10r 1r"() -> (w5738:bool[])
                        n2236 = Index Array(array=w5738, index=0) -> (element=w5736:bool)
                        n2237 = case shown="False" w5736 {
                          tunnel: w5735 -> [_ w5745]
                          frame False {
                            n2238 = local write "Denge Seçimi"(u8 2 ("Denge Seçimi")) -> ()
                            n2239 = local write "count meas"(u16 0 ("count meas")) -> ()
                            n2240 = local write "10R switch"(TRUE ("10R switch")) -> ()
                            n2241 = local write "Boolean 3"(TRUE ("Boolean 4")) -> ()
                            n2242 = local write "PASS 1R"(FALSE ("PASS 1R")) -> ()
                          }
                          frame True {
                            n2243 = local write "Denge Seçimi"(w5745) -> ()
                            n2244 = local write "kelvin switch"(TRUE ("10R switch")) -> ()
                            n2245 = local write "count meas"(u16 0 ("count meas")) -> ()
                            n2246 = local write "Boolean 3"(TRUE ("Boolean 4")) -> ()
                            n2247 = local write "PASS 1R"(FALSE ("PASS 1R")) -> ()
                          }
                        }
                      }
                    }
                    n2248 = case shown="True" w5723 {
                      tunnel: w5722 -> [_ w5733]
                      frame False {
                      }
                      frame True {
                        n2249 = local write "reset values"(TRUE ("reset values")) -> ()
                        n2250 = local write "end time"(w5733) -> ()
                        n2251 = local write "Boolean 3"(TRUE ("Boolean 4")) -> ()
                        n2252 = local write "PASS 1R"(FALSE ("PASS 1R")) -> ()
                      }
                    }
                    n2253 = case shown="True" w5721 {
                      frame False {
                      }
                      frame True {
                        n2254 = local write "RESET SENS X 3"(TRUE ("RESET SENS X 4")) -> ()
                        n2255 = local write "PASS 1R"(FALSE ("PASS 1R")) -> ()
                      }
                    }
                  }
                  frame #3 {
                  }
                }
              }
            }
            n2256 = case shown="True" "auto phase 1R" {
              frame False {
              }
              frame True {
                n2257 = flat-sequence {
                  frame #0 {
                    n2258 = local read "GPIB In"() -> (w5754:refnum<visa-resource-name>)
                    n2259 = call "reference phase.vi"("Reference Phase (0.000 degrees)"="0", "VISA resource name"=w5754) -> ()  [unwired: 8 in, 2 out]
                  }
                  frame #1 {
                    w5756 = u16 0 items=["100 nV", "200 nV", "500 nV", "1 uV", "2 uV", "5 uV", "10 uV", "20 uV", "50 uV", "100 uV", "200 uV", "500 uV", "1 mV"] ("Min. Hassasiyet")
                    n2260 = local read "GPIB In"() -> (w5757:refnum<visa-resource-name>)
                    n2261 = local read "X Range 1R"() -> (w5755:dbl)
                    n2262 = call "GAIN BASIC.vi"("SR850 GPIB In"=w5757, "Max. Hassasiyet"=w5755, "Auto Gain (False)"=FALSE, "Min. Hassasiyet"=w5756) -> ()  [unwired: 10 in, 2 out]
                  }
                  frame #2 {
                    n2263 = local read "X 1.input 1R"() -> (w5759:dbl)
                    n2264 = global write "DB_Global_4_kart-Test.vi" "amplitude 3/1"(w5759) -> ()
                    n2265 = global write "DB_Global_4_kart-Test.vi" "phase 3/1"(w5759) -> ()
                  }
                  frame #3 {
                    n2266 = Wait (ms)(milliseconds to wait=u32 750) -> ()  [unwired: 1 out]
                  }
                  frame #4 {
                    n2267 = local write "read x1 y1 3"(TRUE ("output x")) -> ()
                    n2268 = local write "auto phase 1R"(FALSE ("auto phase wagner")) -> ()
                  }
                }
              }
            }
            n2269 = case shown="True" "RANGE KONTROL X 3" {
              frame False {
              }
              frame True {
                n2270 = local read "Output Denge Kosulu x1_x2"() -> (w5605:dbl[][])
                n2271 = local read "iterasyon 1R"() -> (w5604:dbl)
                n2272 = local read "frekans index"() -> (w5597:dbl)
                n2273 = local read "input 1 x [1R]"() -> (w5606:dbl)
                n2274 = local read "input 2 x [1R]"() -> (w5607:dbl)
                n2275 = local read "output 2 x [1R]"() -> (w5601:dbl)
                n2276 = local read "output 1 x [1R]"() -> (w5603:dbl)
                n2277 = call "Range Kontrol X.vi"("denge degeri"=3.0, "iterasyon Denge"=w5604, "frekans index"=w5597, "Denge Kosulu x1_x2"=w5605, "Xk"=w5606, "X(k-1)"=w5607, "output x 1"=w5603, "output x 2"=w5601) -> ("Output X(k-1)"=w5596:dbl, "result output x"=w5608:dbl, "KONTROL Y"=w5600:bool, "IF ELSE"=w5599:bool, "Start Denge Y"=w5598:bool)  [unwired: 7 in]
                n2278 = local write "1R X(k-1)"(w5596) -> ()
                n2279 = local write "result output x [1R]"(w5608) -> ()
                n2280 = flat-sequence {
                  tunnel: w5600 -> [w5611]
                  tunnel: w5599 -> [w5610]
                  tunnel: w5598 -> [w5609]
                  frame #0 {
                    n2281 = case shown="True" w5609 {
                      frame False {
                      }
                      frame True {
                        n2282 = local write "Start 1R Y"(TRUE ("Start Wagner Y")) -> ()
                      }
                    }
                    n2283 = case shown="True" w5610 {
                      frame False {
                      }
                      frame True {
                        n2284 = local write "IF ELSE X 3"(TRUE ("IF ELSE X 4")) -> ()
